vi "IntializeBallSystem.vi"   [LabVIEW 2019]
uses:
  <vilib>/Rock Robotics/SystemInterfaces/DIO/FPGA_DIOPWMChannel.ctl
  <vilib>/Rock Robotics/WPI/Solenoid/WPI_SolenoidChannel.ctl
  <vilib>/Rock Robotics/WPI/MotorControl/WPI_MotorControlOpen Talon.vi
  <vilib>/Rock Robotics/WPI/Solenoid/WPI_SolenoidOpenSingle.vi
types:
  T1 = typedef "FPGA_DIOPWMChannel.ctl" = enum8{"PWM 0", "PWM 1", "PWM 2", "PWM 3", "PWM 4", "PWM 5", "PWM 6", "PWM 7", "PWM 8", "PWM 9", "PWM MXP 0", "PWM MXP 1", "PWM MXP 2", "PWM MXP 3", "PWM MXP 4", "PWM MXP 5", "PWM MXP 6", "PWM MXP 7", "PWM MXP 8", "PWM MXP 9", "Invalid"}
  T2 = typedef "WPI_SolenoidChannel.ctl" = enum8{"Solenoid 0", "Solenoid 1", "Solenoid 2", "Solenoid 3", "Solenoid 4", "Solenoid 5", "Solenoid 6", "Solenoid 7", "Invalid"}
  T3 = typedef "WPI_SolenoidDevRef.ctl" = cluster{"DevStatus":errorcluster, "Pneumatics Control Module":u8, "Forward Solenoid Channel":T2, "Reverse Solenoid Channel":T2}
  T4 = typedef "WPI_MotorControlDeviceRef.ctl" = cluster{"DeviceStatus":errorcluster, "Type":T5, "PWM":cluster{"PWM Channel":T1, "DeadBand":T6}, "CAN":cluster{"Device Number":u8, "SetOutput VI Ref":variant, "GetOutput VI Ref":variant, "Enable VI Ref":variant, "Disable VI Ref":variant, "Data":variant}, "Invert":bool, "DIO PWM":cluster{"PWM \"Enable\" Channel":T1, "DIOChannel":T7, "PWM Rate":dbl}}
  T5 = typedef "WPI_MotorControlType.ctl" = enum16{"PWM", "CAN", "DIO PWM"}
  T6 = typedef "WPI_PWMDeadband.ctl" = cluster{"Name":string, "maxPositivePwm":i32, "minPositivePwm":i32, "centerPwm":i32, "maxNegativePwm":i32, "minNegativePwm":i32, "angularRange":u16}
  T7 = typedef "FPGA_DIOChannel.ctl" = enum8{"DIO 0", "DIO 1", "DIO 2", "DIO 3", "DIO 4", "DIO 5", "DIO 6", "DIO 7", "DIO 8", "DIO 9", "DIO MXP 0", "DIO MXP 1", "DIO MXP 2", "DIO MXP 3", "DIO MXP 4", "DIO MXP 5", "DIO MXP 6", "DIO MXP 7", "DIO MXP 8", "DIO MXP 9", "DIO MXP 10", "DIO MXP 11", "DIO MXP 12", "DIO MXP 13", "DIO MXP 14", "DIO MXP 15", "SPI Port CS1", "SPI Port CS2", "SPI Port CS3", "SPI Port MISO", "SPI Port MOSI", "Invalid"}
  T8 = typedef "WPI_CameraDevRef.ctl" = cluster{"Camera Address":string, "CameraStatus":errorcluster}
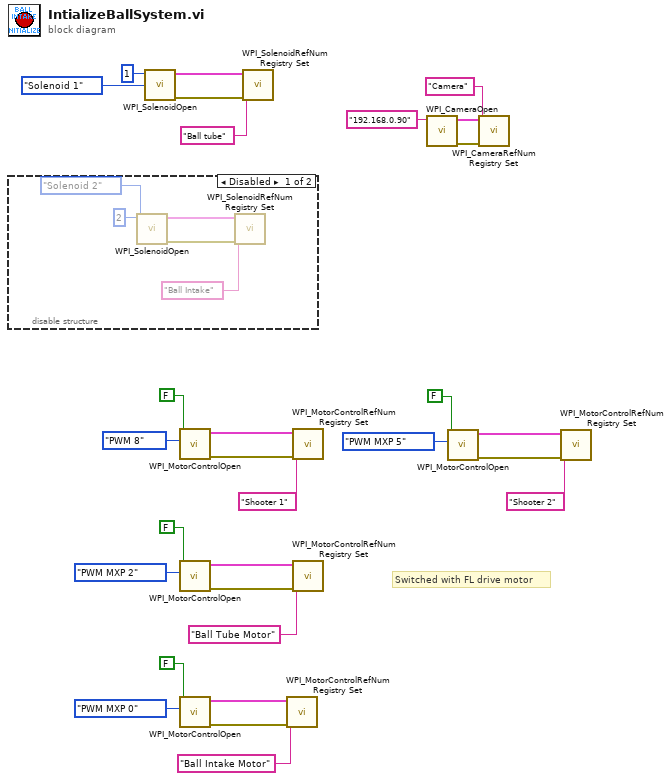
[diagram p0: block diagram]
diagram:
  # "Switched with FL drive motor"
  n1 = disable-structure shown="Disabled" {
    frame Disabled {
      n2 = call-poly <vilib>:"WPI_SolenoidOpen.vi"("Solenoid Channel"=WPI_SolenoidChannel."Solenoid 2", "Pneumatics Control Module (0)"=u8 2) -> ("error out"=w34:errorcluster, "SolenoidDevRef"=w33:T3)  [unwired: 8 in]
      n3 = call <vilib>:"WPI_SolenoidRefNum Registry Set.vi"("error in (no error)"=w34, "refnum name"="Ball Intake", "SolenoidDevRef"=w33) -> ()  [unwired: 7 in, 2 out]
    }
    frame Enabled {
    }
  }
  n4 = call-poly <vilib>:"WPI_SolenoidOpen.vi"("Solenoid Channel"=WPI_SolenoidChannel."Solenoid 1", "Pneumatics Control Module (0)"=u8 1) -> ("error out"=w13:errorcluster, "SolenoidDevRef"=w14:T3)  [unwired: 8 in]
  n5 = call-poly <vilib>:"WPI_MotorControlOpen.vi"("Eliminate Deadband"=FALSE, "PWM Channel"=FPGA_DIOPWMChannel."PWM 8") -> ("error out"=w28:errorcluster, "MotorControlDeviceRef"=w29:T4)  [unwired: 8 in]
  n6 = call-poly <vilib>:"WPI_MotorControlOpen.vi"("Eliminate Deadband"=FALSE, "PWM Channel"=FPGA_DIOPWMChannel."PWM MXP 2") -> ("error out"=w22:errorcluster, "MotorControlDeviceRef"=w21:T4)  [unwired: 8 in]
  n7 = call-poly <vilib>:"WPI_MotorControlOpen.vi"("Eliminate Deadband"=FALSE, "PWM Channel"=FPGA_DIOPWMChannel."PWM MXP 0") -> ("error out"=w19:errorcluster, "MotorControlDeviceRef"=w20:T4)  [unwired: 8 in]
  n8 = call <vilib>:"WPI_SolenoidRefNum Registry Set.vi"("error in (no error)"=w13, "refnum name"="Ball tube", "SolenoidDevRef"=w14) -> ()  [unwired: 7 in, 2 out]
  n9 = call <vilib>:"WPI_MotorControlRefNum Registry Set.vi"("error in (no error)"=w19, "refnum name"="Ball Intake Motor", "MotorControlDevRef"=w20) -> ()  [unwired: 7 in, 2 out]
  n10 = call <vilib>:"WPI_MotorControlRefNum Registry Set.vi"("error in (no error)"=w28, "refnum name"="Shooter 1", "MotorControlDevRef"=w29) -> ()  [unwired: 7 in, 2 out]
  n11 = call <vilib>:"WPI_MotorControlRefNum Registry Set.vi"("error in (no error)"=w22, "refnum name"="Ball Tube Motor", "MotorControlDevRef"=w21) -> ()  [unwired: 7 in, 2 out]
  n12 = call <vilib>:"WPI_CameraOpen.vi"("Camera Address"="192.168.0.90") -> ("error out"=w9:errorcluster, "CameraDevRef"=w8:T8)  [unwired: 9 in]
  n13 = call-poly <vilib>:"WPI_MotorControlOpen.vi"("Eliminate Deadband"=FALSE, "PWM Channel"=FPGA_DIOPWMChannel."PWM MXP 5") -> ("error out"=w2:errorcluster, "MotorControlDeviceRef"=w1:T4)  [unwired: 8 in]
  n14 = call <vilib>:"WPI_CameraRefNum Registry Set.vi"("error in (no error)"=w9, "refnum name"="Camera", "CameraDevRef"=w8) -> ()  [unwired: 7 in, 2 out]
  n15 = call <vilib>:"WPI_MotorControlRefNum Registry Set.vi"("error in (no error)"=w2, "refnum name"="Shooter 2", "MotorControlDevRef"=w1) -> ()  [unwired: 7 in, 2 out]
